vi "SampleDependentVI.vi"(8 "error in (no error)":errorcluster, 11 "SampleDependentClass in":refnum<class "SampleDependentClass.lvclass">) -> (0 "error out":errorcluster, 3 "SampleDependentClass out":refnum<class "SampleDependentClass.lvclass">)   [LabVIEW 2019, in "SampleDependentLib.lvlib" / "SampleDependentClass.lvclass"]
uses:
  SampleDependentClass.lvclass
  <vilib>/xml/NI_XML.lvlib
  <vilib>/xml/Load XML File.vi
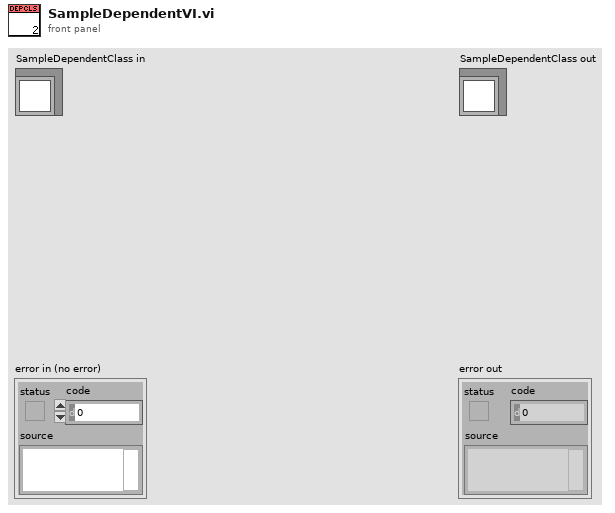
[diagram p1: front panel]
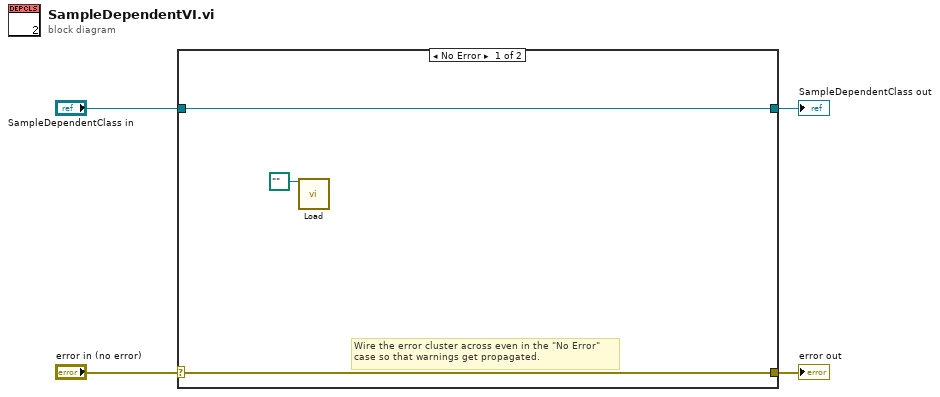
[diagram p0: block diagram]
diagram:
  n1 = case shown="No Error" "error in (no error)" {
    selector: "error in (no error)" -> [w6 w9]
    tunnel: [w6 w9] -> w3
    tunnel: [w7 w8] -> w1
    tunnel: "SampleDependentClass in" -> [w7 w8]
    frame No Error {
      # "Wire the error cluster across even in the \"No Error\"\ncase so that warnings get propagated."
      n2 = call-poly <vilib>:"Load.vi"("path to XML document"=path "") -> ()  [unwired: 12 in, 3 out]
    }
    frame Error {
    }
  }
  "error out" <- w3
  "SampleDependentClass out" <- w1
